vi "Dynamixel XL320 Move Motor.vi"() -> ()   [LabVIEW 2017]
uses:
  Users/Pierre-Olivier/Desktop/Projet MAKI/makiprog_2015/Poubelle/Register_Write_R16/C/Program Files (x86)/National Instruments/LabVIEW 2017/instr.lib/Dynamixel XL320/Public/Motor Operation/Low Level/XL320_Baud Setting.ctl
  Users/Pierre-Olivier/Desktop/Projet MAKI/makiprog_2015/Poubelle/Register_Write_R16/C/Program Files (x86)/National Instruments/LabVIEW 2017/instr.lib/Dynamixel XL320/Dynamixel XL320.lvlib
panel:
  in  "Baud rate (1,000,000 bps)":T1=3 items=["9600 bps", "57600 bps", "115200 bps", "1,000,000 bps"]
  out "Command to Serial":string
  in  "Goal Speed (RPM)":dbl(knob)=40.0 min=0.0 max=114.0 step=1.0 scale=0.0..114.0
  in  "Goal Position (150 deg)":dbl(knob)=150.0 min=0.0 max=300.0 step=1.0 scale=0.0..300.0
  in  "Motor ID (5)":u8=5
  out "error out":errorcluster
  in  "stop":bool
  in  "VISA resource name":refnum<visa-resource-name>
  # "Ghislain REMY, IUT de Cachan, 2015 December 2015"
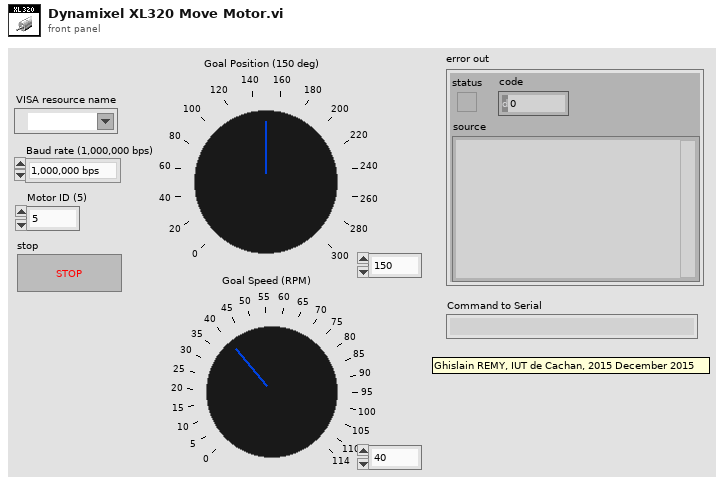
[diagram p1: front panel]
types:
  T1 = typedef "Dynamixel XL320.lvlib/XL320_Baud Setting.ctl" = u8
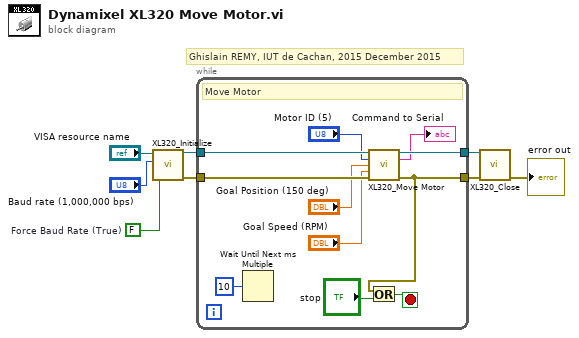
[diagram p0: block diagram]
diagram:
  w1 = FALSE  # Force Baud Rate (True)
  # "Ghislain REMY, IUT de Cachan, 2015 December 2015"
  n1 = call "XL320_Initialize.vi"("Force Baud Rate (True)"=w1, "Baud rate (1,000,000 bps)"="Baud rate (1,000,000 bps)", "VISA resource name"="VISA resource name") -> ("error out"=w4:errorcluster, "VISA resource name out"=w7:refnum<visa-resource-name>)  [unwired: 7 in]
  n2 = while {
    tunnel: w7 -> [w19]
    tunnel: [w18] -> w6
    tunnel: [w11] -> w5
    tunnel: w4 -> [w17]
    stop <- w13 stop-if-true
    # "Move Motor"
    n3 = Wait Until Next ms Multiple(millisecond multiple=u32 10) -> ()  [unwired: 1 out]
    n4 = call "XL320_Move Motor.vi"("VISA resource name"=w19, "Motor ID (0)"="Motor ID (5)", "Goal Position (150 deg)"="Goal Position (150 deg)", "Goal Speed (RPM)"="Goal Speed (RPM)", "error in (no error)"=w17) -> ("VISA resource name out"=w18:refnum<visa-resource-name>, "Command to Serial"=→"Command to Serial":string, "error out"=w11:errorcluster)  [unwired: 8 in]
    n5 = Or(x=w11, y="stop") -> (x .or. y?=w13:bool)
  }
  n6 = call "XL320_Close.vi"("error in (no error)"=w5, "VISA resource name"=w6) -> ("error out"=→"error out":errorcluster)  [unwired: 9 in]
